vi "gantry_feedback_control.vi"(6 "VISA resource name":refnum<visa-resource-name>, 8 "current motor speed":string, 9 "Images completed":dbl, 10 "Default microcontroller clockrate":dbl=165.0, 11 "Wheel Position (abs)":dbl) -> (0 "read inc/dec motor speed":string="0", 4 "VISA resource name out":refnum<visa-resource-name>)   [LabVIEW 2021]
panel:
  in  "limit on speed inc/dec":dbl=2.0 format="%#_13g"
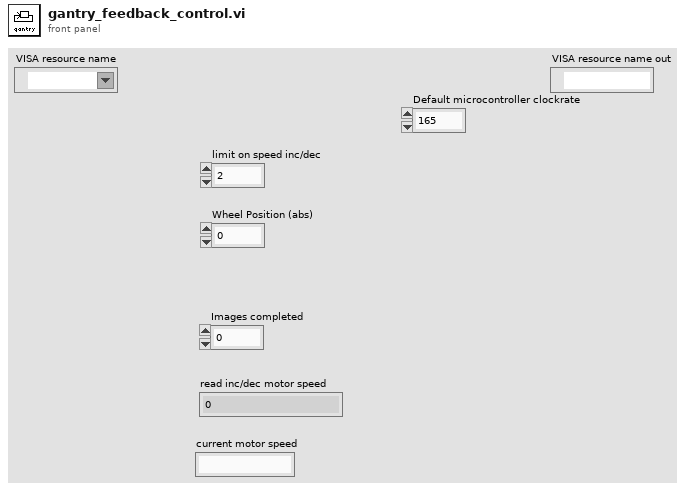
[diagram p1: front panel]
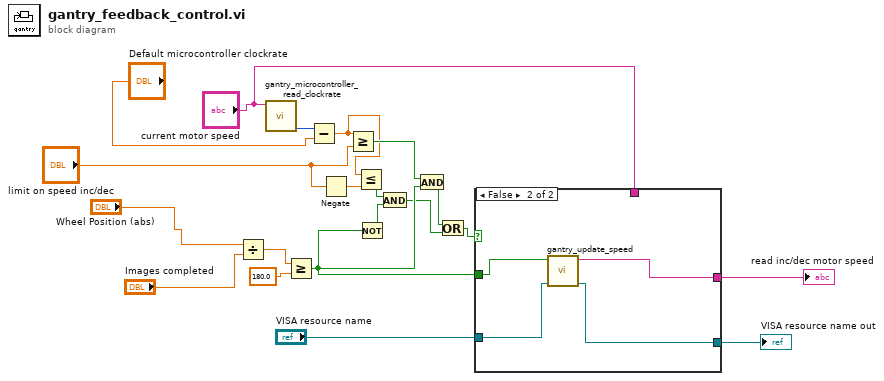
[diagram p0: block diagram]
diagram:
  n1 = Divide(x="Wheel Position (abs)", y="Images completed") -> (x/y=w20:dbl)
  n2 = call "gantry_microcontroller_read_clockrate.vi"("read inc/dec motor speed"="current motor speed") -> ("number"=w17:i32)  [unwired: 10 in]
  n3 = Greater Or Equal?(x=w20, y=180.0) -> (x >= y?=w10:bool)
  n4 = Subtract(x=w17, y="Default microcontroller clockrate") -> (x-y=w15:dbl)
  n5 = Negate(x="limit on speed inc/dec") -> (-x=w13:dbl)
  n6 = Greater Or Equal?(x=w15, y="limit on speed inc/dec") -> (x >= y?=w16:bool)
  n7 = Less Or Equal?(x=w15, y=w13) -> (x <= y?=w12:bool)
  n8 = Not(x=w10) -> (.not. x?=w11:bool)
  n9 = And(x=w12, y=w11) -> (x .and. y?=w9:bool)
  n10 = And(x=w16, y=w10) -> (x .and. y?=w8:bool)
  n11 = Or(x=w8, y=w9) -> (x .or. y?=w7:bool)
  n12 = case shown="False" w7 {
    tunnel: w10 -> [_ w26]
    tunnel: [w22 w25] -> w6
    tunnel: "current motor speed" -> [w22 _]
    tunnel: "VISA resource name" -> [w21 w24]
    tunnel: [w21 w23] -> w1
    frame True {
      # "don't keep going slower"
    }
    frame False {
      n13 = call "gantry_update_speed.vi"("VISA resource name"=w24, "inc/dec"=w26) -> ("VISA resource name out"=w23:refnum<visa-resource-name>, "read buffer"=w25:string)  [unwired: 8 in]
    }
  }
  "read inc/dec motor speed" <- w6
  "VISA resource name out" <- w1
